vi "MarkerImage.vi"(5 "Disabled":bool, 6 "error in":errorcluster, 9 "knob":refnum<vi>) -> (0 "error out":errorcluster, 3 "knob reference out":refnum<vi>, 4 "marker":T1)   [LabVIEW 2014, in "Knob.lvclass"]
uses:
  Knob.lvclass
  <vilib>/picture/picture.llb/imagedata.ctl
  <vilib>/Utility/miscctls.llb/LVForegroundBackgroundColorsTypeDef.ctl
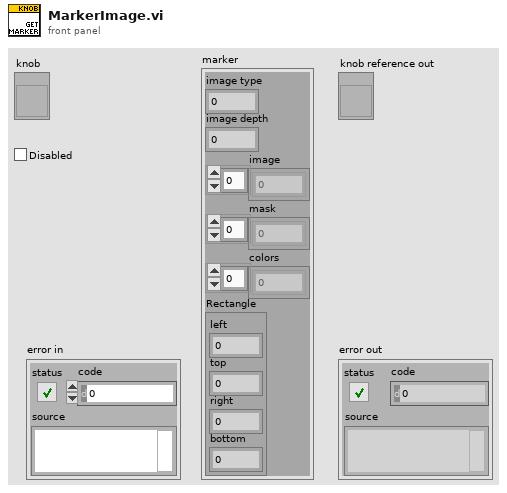
[diagram p1: front panel]
types:
  T1 = typedef "imagedata.ctl" = cluster{"image type":i32, "image depth":i32, "image":u8[], "mask":u8[], "colors":u32[], "Rectangle":cluster{"left":i16, "top":i16, "right":i16, "bottom":i16}}
  T2 = enum8{"Enabled", "Disabled", "Disabled and Grayed Out"}
  T3 = typedef "LVForegroundBackgroundColorsTypeDef.ctl" = cluster{"Foreground Color":u32, "Background Color":u32}
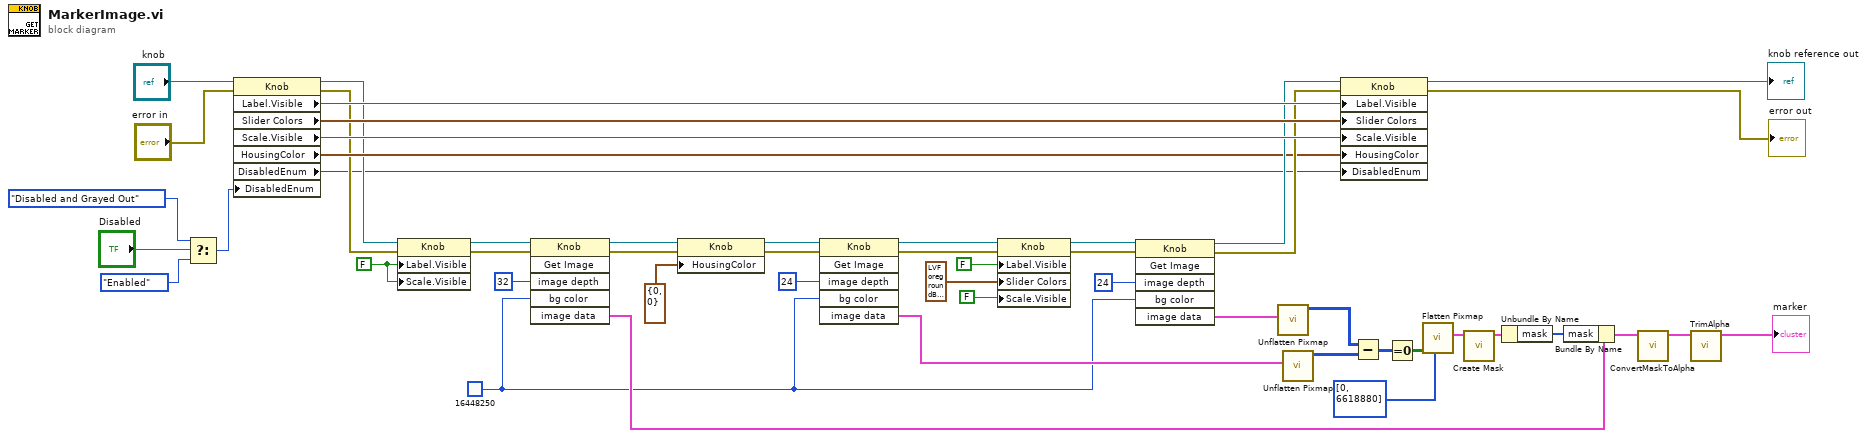
[diagram p0: block diagram]
diagram:
  w11 = u32 16448250
  w36 = FALSE ("Label.Visible")
  n1 = Select(t=T2."Disabled and Grayed Out" ("Disabled"), s="Disabled", f=T2."Enabled") -> (s? t:f=w2:T2)
  n2 = property on="Property Node" class="Knob"(reference="knob", error in="error in", "DisabledEnum"=w2) -> (reference out=w21:refnum<vi>, error out=w20:errorcluster, "Label.Visible"=w50:bool, "Slider Colors"=w48:T3, "Scale.Visible"=w49:bool, "HousingColor"=w35:T3, "DisabledEnum"=w1:T2)
  n3 = property on="Property Node" class="Knob"(reference=w21, error in=w20, "Label.Visible"=w36, "Scale.Visible"=w36) -> (reference out=w24:refnum<vi>, error out=w23:errorcluster)
  n4 = invoke class="Knob" method="Get Image"(reference=w24, error in=w23, "image depth"=32 ("Image Depth"), "bg color"=w11) -> (reference out=w19:refnum<vi>, error out=w18:errorcluster, "image data"=w14:T1)  [unwired: 2 in, 3 out]
  n5 = property on="Property Node" class="Knob"(reference=w19, error in=w18, "HousingColor"=T3 {"Foreground Color"=0, "Background Color"=0} ("Slider Colors")) -> (reference out=w17:refnum<vi>, error out=w16:errorcluster)
  n6 = invoke class="Knob" method="Get Image"(reference=w17, error in=w16, "image depth"=24 ("Image Depth"), "bg color"=w11) -> (reference out=w40:refnum<vi>, error out=w41:errorcluster, "image data"=w34:T1)  [unwired: 2 in, 3 out]
  n7 = property on="Property Node" class="Knob"(reference=w40, error in=w41, "Label.Visible"=FALSE, "Slider Colors"=T3 {"Foreground Color"=16777216, "Background Color"=16777216}, "Scale.Visible"=FALSE ("Label.Visible")) -> (reference out=w45:refnum<vi>, error out=w46:errorcluster)
  n8 = invoke class="Knob" method="Get Image"(reference=w45, error in=w46, "image depth"=24 ("Image Depth"), "bg color"=w11) -> (reference out=w39:refnum<vi>, error out=w38:errorcluster, "image data"=w27:T1)  [unwired: 2 in, 3 out]
  n9 = call <vilib>:"Unflatten Pixmap.vi"("image data"=w27) -> ("24-bit pixmap"=w33:u32[][])  [unwired: 4 in, 6 out]
  n10 = call <vilib>:"Unflatten Pixmap.vi"("image data"=w34) -> ("24-bit pixmap"=w32:u32[][])  [unwired: 4 in, 6 out]
  n11 = property on="Property Node" class="Knob"(reference=w39, error in=w38, "Label.Visible"=w50, "Slider Colors"=w48, "Scale.Visible"=w49, "HousingColor"=w35, "DisabledEnum"=w1) -> (reference out=→"knob reference out":refnum<vi>, error out=→"error out":errorcluster)
  n12 = Subtract(x=w33, y=w32) -> (x-y=w31:u32[][])
  n13 = Equal To 0?(x=w31) -> (x = 0?=w30:bool[][])
  n14 = call <vilib>:"Flatten Pixmap.vi"("colors"=u32[] [0, 6618880], "1-bit pixmap"=w30) -> ("image data"=w28:T1)  [unwired: 9 in]
  n15 = call <vilib>:"Create Mask.vi"("image data"=w28) -> ("image data"=w26:T1)  [unwired: 10 in]
  n16 = Unbundle By Name(w26) -> ("mask"=w25:u8[])
  n17 = Bundle By Name(cluster=w14, "mask"=w25) -> (w13:T1)
  n18 = call "ConvertMaskToAlpha.vi"("input cluster"=w13) -> ("output cluster"=w12:T1)  [unwired: 10 in]
  n19 = call "TrimAlpha.vi"("input cluster"=w12) -> ("output cluster"=→"marker":T1)  [unwired: 10 in]
